vi "Get Popcorn Shot.vi"(9 "Input Velocities":T1, 10 "Y Pressed?":bool, 11 "B Pressed?":bool) -> (1 "Transfer":dbl, 2 "Hood":dbl, 3 "RPM":dbl)   [LabVIEW 2025]
uses:
  swerve-template/Type Definitions/Data/Robot Velocities.ctl
panel:
  in  "Popcorn Default Hood":dbl=19.0
  in  "Popcorn Default Vel":dbl=700.0
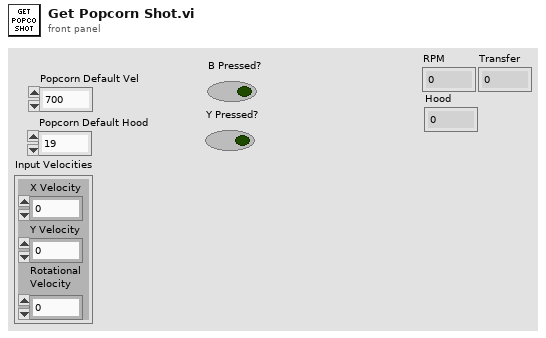
[diagram p1: front panel]
types:
  T1 = typedef "Robot Velocities.ctl" = cluster{"X Velocity":dbl, "Y Velocity":dbl, "Rotational \nVelocity":dbl}
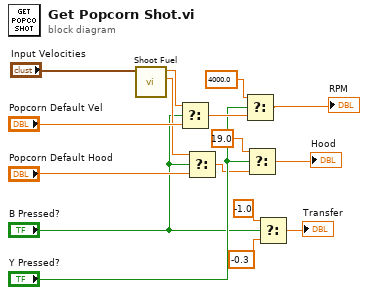
[diagram p0: block diagram]
diagram:
  n1 = call "Shoot Fuel.vi"("Input Velocities"="Input Velocities") -> ("Hood Setpoint"=w12:dbl, "Shooter RPM"=w15:dbl)  [unwired: 9 in]
  n2 = Select(t=w15, s="B Pressed?", f="Popcorn Default Vel") -> (s? t:f=w11:dbl)
  n3 = Select(t=w12, s="B Pressed?", f="Popcorn Default Hood") -> (s? t:f=w8:dbl)
  n4 = Select(t=4000.0 ("Hoard Shot Velocity"), s="Y Pressed?", f=w11) -> (s? t:f=→"RPM":dbl)
  n5 = Select(t=19.0 ("Hoard Hood Setpoint"), s="Y Pressed?", f=w8) -> (s? t:f=→"Hood":dbl)
  n6 = Select(t=-1.0, s="B Pressed?", f=-0.3) -> (s? t:f=→"Transfer":dbl)
